vi "EJEM18.vi"() -> ()   [LabVIEW 2013]
panel:
  out "Array 3":dbl[](array[numeric])
  in  "length":i32
  in  "index":i32
  out "Array 2":dbl[](array[numeric])
  in  "y":dbl
  out "Array":dbl[](array[numeric])
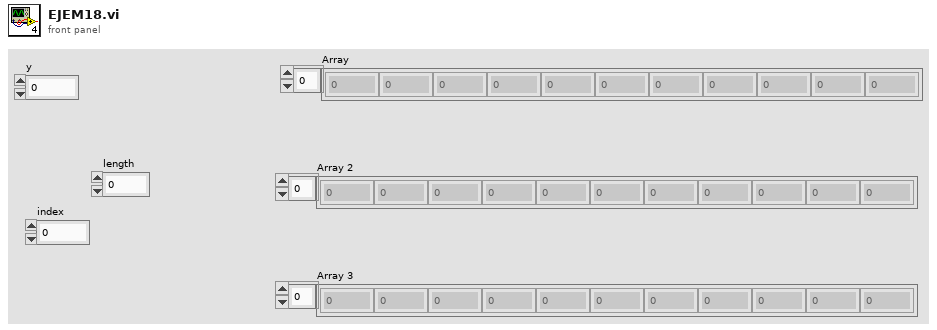
[diagram p1: front panel]
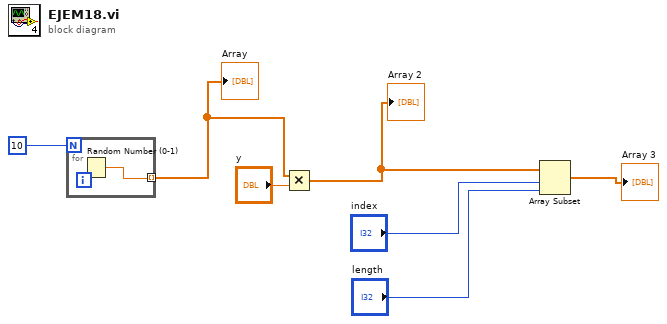
[diagram p0: block diagram]
diagram:
  n1 = for {
    N: 10 -> [_]
    tunnel: [w8] -> w5 mode=indexing
    n2 = Random Number (0-1)() -> (number: 0 to 1=w8:dbl)
  }
  "Array" <- w5
  n3 = Multiply(x=w5, y="y") -> (x*y=w4:dbl[])
  "Array 2" <- w4
  n4 = Array Subset(array=w4, index="index", length="length") -> (→"Array 3":dbl[])
